vi "test_TCP_2_parseRead_p2.vi"(9 "input_arrayIndices":u16[](array[numeric]), 11 "input_stringAccum":string) -> (2 "output_value":i32, 3 "output_stringValue":string)   [LabVIEW 2014]
panel:
  out "x = y?":bool
  out "substring 2":string
  out "substring":string
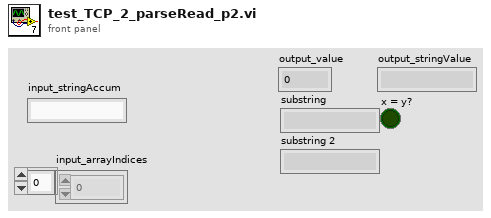
[diagram p1: front panel]
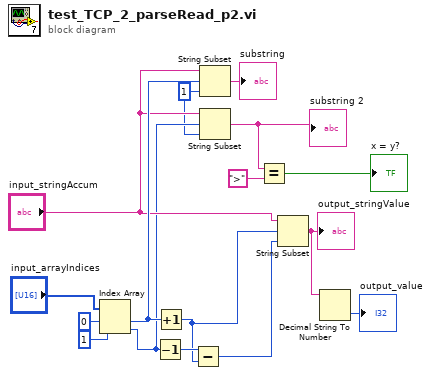
[diagram p0: block diagram]
diagram:
  w5 = 1 ("length (rest)")
  n1 = Index Array(array="input_arrayIndices", index #1=0 ("index"), index #2=1 ("index")) -> (element #1=w8:u16, element #2=w6:u16)
  n2 = Decrement(x=w6) -> (x-1=w13:u16)
  n3 = Increment(x=w8) -> (x+1=w12:u16)
  n4 = Subtract(x=w13, y=w12) -> (x-y=w9:u16)
  n5 = String Subset(string="input_stringAccum", offset (0)=w8, length (rest)=w5) -> (substring=→"substring":string)
  n6 = String Subset(string="input_stringAccum", offset (0)=w6, length (rest)=w5) -> (substring=w2:string)
  "substring 2" <- w2
  n7 = Equal?(x=w2, y=">") -> (x = y?=→"x = y?":bool)
  n8 = String Subset(string="input_stringAccum", offset (0)=w12, length (rest)=w9) -> (substring=w11:string)
  "output_stringValue" <- w11
  n9 = Decimal String To Number(string=w11) -> (number=→"output_value":i32)  [unwired: 2 in, 1 out]
